vi "FROG_RMSerror.vi"(4 "Experiment Trace":dbl[][](array[numeric]), 5 "Fit Trace":dbl[][](array[numeric])) -> (0 "Histogram RMS Error":dbl, 1 "FFT RMS Error":dbl, 2 "RMS Error":dbl)   [LabVIEW 2013]
uses:
  <vilib>/Analysis/2dsp.llb/2D Real FFT.vi
  <vilib>/Analysis/baseanly.llb/Quick Scale 2D.vi
  <vilib>/Analysis/NI_AALBase.lvlib
  <vilib>/Analysis/NI_AALPro.lvlib
panel:
  out "Fit Trace Historgram":i32[][](graph)
  out "Experiment Trace Histogram":i32[][](graph)
  out "Error Log":dbl[](graph)
  out "Fit Trace FFT":dbl[][](graph)
  out "Experiment Trace FFT":dbl[][](graph)
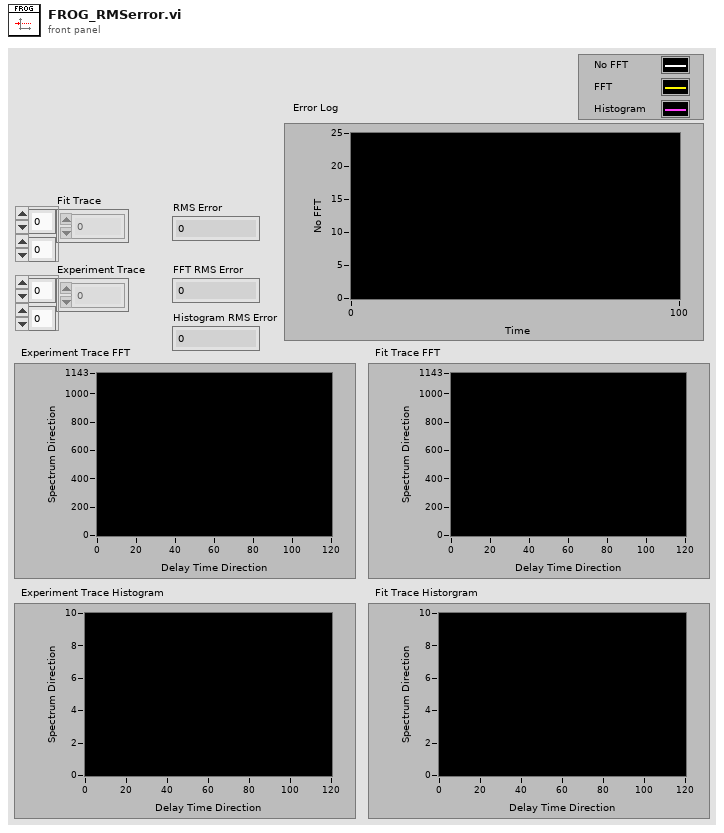
[diagram p1: front panel]
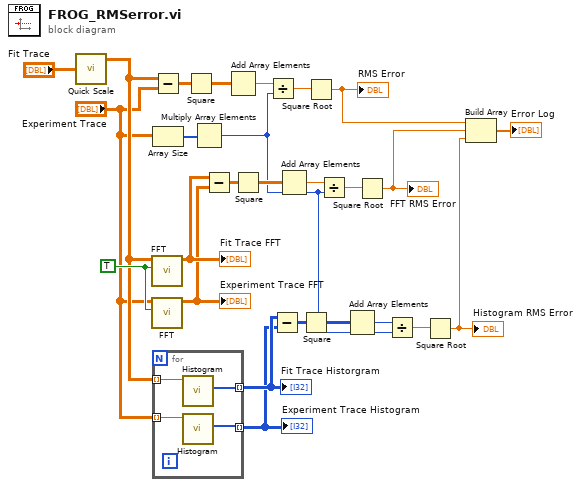
[diagram p0: block diagram]
diagram:
  w20 = TRUE ("shift?")
  n1 = call-poly <vilib>:"Quick Scale.vi"("X"="Fit Trace") -> ("Yij=Xij/Max|X|"=w10:dbl[][])  [unwired: 2 out]
  n2 = call-poly <vilib>:"FFT.vi"("shift?"=w20, "X"=w10) -> ("FFT {X}"=w15:cdb[][])  [unwired: 8 in, 1 out]
  "Fit Trace FFT" <- w15
  n3 = call-poly <vilib>:"FFT.vi"("shift?"=w20, "X"="Experiment Trace") -> ("FFT {X}"=w14:cdb[][])  [unwired: 8 in, 1 out]
  "Experiment Trace FFT" <- w14
  n4 = Subtract(x=w10, y="Experiment Trace") -> (x-y=w22:dbl[][])
  n5 = Array Size(array="Experiment Trace") -> (size(s)=w25:i32[])
  n6 = for {
    tunnel: w10 -> [w30] mode=indexing
    tunnel: "Experiment Trace" -> [w29] mode=indexing
    tunnel: [w28] -> w4 mode=indexing
    tunnel: [w27] -> w3 mode=indexing
    n7 = call <vilib>:"Histogram.vi"("X"=w30) -> ("Histogram: h(x)"=w28:i32[])  [unwired: 7 in, 3 out]
    n8 = call <vilib>:"Histogram.vi"("X"=w29) -> ("Histogram: h(x)"=w27:i32[])  [unwired: 7 in, 3 out]
  }
  "Experiment Trace Histogram" <- w3
  "Fit Trace Historgram" <- w4
  n9 = Square(x=w22) -> (x^2=w23:dbl[][])
  n10 = Multiply Array Elements(1:w25) -> (0:w2:i32)
  n11 = Subtract(x=w15, y=w14) -> (x-y=w17:cdb[][])
  n12 = Add Array Elements(numeric array=w23) -> (sum=w21:dbl)
  n13 = Square(x=w17) -> (x^2=w18:cdb[][])
  n14 = Divide(x=w21, y=w2) -> (x/y=w26:dbl)
  n15 = Subtract(x=w4, y=w3) -> (x-y=w6:i32[][])
  n16 = Add Array Elements(numeric array=w18) -> (sum=w16:cdb)
  n17 = Square(x=w6) -> (x^2=w7:i32[][])
  n18 = Square Root(x=w26) -> (sqrt(x)=w13:dbl)
  "RMS Error" <- w13
  n19 = Divide(x=w16, y=w2) -> (x/y=w19:cdb)
  n20 = Add Array Elements(numeric array=w7) -> (sum=w5:i32)
  n21 = Square Root(x=w19) -> (sqrt(x)=w12:cdb)
  "FFT RMS Error" <- w12
  n22 = Divide(x=w5, y=w2) -> (x/y=w8:dbl)
  n23 = Square Root(x=w8) -> (sqrt(x)=w1:dbl)
  "Histogram RMS Error" <- w1
  n24 = Build Array(w13, w12, w1) -> (→"Error Log":cdb[])
